vi "I am alive.vi"(8 "error in (no error)":errorcluster, 11 "Guardian in":refnum<class "Guardian.lvclass">) -> (0 "error out":errorcluster, 3 "Guardian out":refnum<class "Guardian.lvclass">)   [LabVIEW 2026, in "TALOS.lvlib" / "Guardian.lvlib" / "Guardian.lvclass"]
doc: "This VI updates the Guardian Health SV, indicating the Guardian is working properly to the other Guardians."
uses:
  Guardian.lvclass
  C:/LabVIEW Code/TALOS/builds/Actor Framework PPL/Actor Framework.lvlibp/1abvi3w/vi.lib/ActorFramework/Actor/Actor.lvclass
  C:/LabVIEW Code/TALOS/talos/Ancestor/Ancestor/Ancestor.lvclass
  Guardian.lvclass/Guardian.ctl
  Ancestor/Ancestor/Ancestor.lvclass/Ancestor.ctl
  Guardian Messages/Message to Other Guardian Msg/Message to Other Guardian Msg.lvclass/Message to Other Guardian Msg.ctl
  Guardian Messages/TCP-SV Message Interpreter Msg/TCP-SV Message Interpreter Msg.lvclass/TCP-SV Message Interpreter Msg.ctl
  Guardian Messages/Message to Other Guardian Msg/Send Message to Other Guardian.vi
  Ancestor/Ancestor/Read ID.vi
  Support VIs/Search Array of Strings.vi
  Guardian Messages/TCP-SV Message Interpreter Msg/Send TCP-SV Message Interpreter.vi
  Support VIs/Substitute Error.vi
  Support VIs/Generate Error.vi
  FGV/Error Memory/Get Error Description.vi
  Support VIs/Get PC name.vi
  Support VIs/Get Class Name.vi
  <vilib>/Utility/error.llb/Clear Errors.vi
  FGV/Error Memory/Error Memory Core.vi
  <vilib>/AdvancedString/Delimited String to 1D String Array.vi
  <vilib>/AdvancedString/Delimited String to 1D String Array (string).vi
  Support VIs/Circus Root Path.vi
  FGV/Error Memory/Error Crt Lvl checker.vi
  FGV/Error Memory/Error Memory Core.vi/40c8088d-b597-4017-91af-faa98e00292e.vi
  FGV/Error Memory/Error Memory Core.vi/d4a3ab98-063c-4e44-b43d-fbdcfe6c2be2.vi
  Support VIs/Global Constants.vi
  Support VIs/Circus Critical PCs List.vi
  builds/Actor Framework PPL/Actor Framework.lvlibp/1abvi3w/vi.lib/ActorFramework/Actor/Read Self Enqueuer.vi
  builds/Actor Framework PPL/Actor Framework.lvlibp/1abvi3w/vi.lib/ActorFramework/Message Enqueuer/Enqueue.vi
  Support VIs/Global Memory.vi
  <vilib>/Utility/LVClass/Get LV Class Name.vi
  Support VIs/Is in Packed Library.vi
  Support VIs/TALOS Root path.vi
  Support VIs/Read CSV worksheet.vi
  <vilib>/Utility/error.llb/General Error Handler.vi
  Support VIs/Error Log.vi
  Guardian Messages/Message to Other Guardian Msg/Message to Other Guardian Msg.lvclass
  Guardian Messages/TCP-SV Message Interpreter Msg/TCP-SV Message Interpreter Msg.lvclass
  Ancestor/Ancestor/Ancestor.lvclass
  <vilib>/Comparison/Equal/Equal Functor/Equal Functor.lvclass
  Classes/Guardian List/Guardian List.lvclass
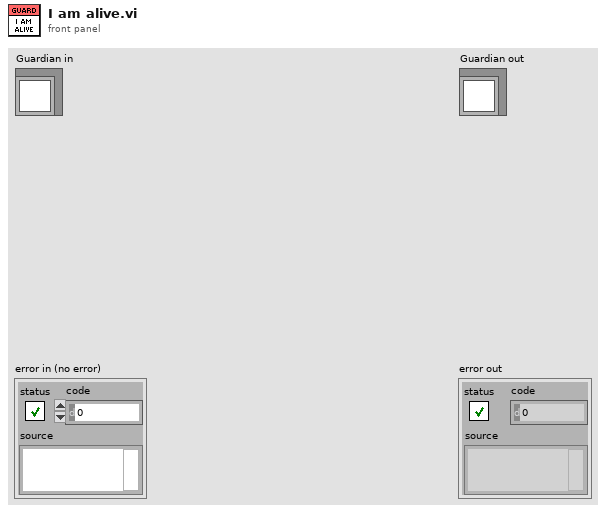
[diagram p1: front panel]
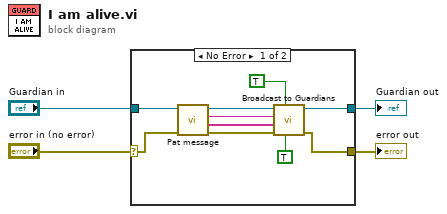
[diagram p0: block diagram]
diagram:
  n1 = case shown="No Error" "error in (no error)" {
    selector: "error in (no error)" -> [w13 w16]
    tunnel: [w8 w16] -> w3
    tunnel: [w9 w15] -> w1
    tunnel: "Guardian in" -> [w14 w15]
    frame No Error {
      n2 = call "Pat message.vi"("error in (no error)"=w13, "Guardian in"=w14) -> ("error out"=w11:errorcluster, "Data"=w10:string[], "Message name"=w6:string, "Guardian out"=w12:refnum<class "Guardian.lvclass">)  [unwired: 6 in]
      n3 = call "Broadcast to Guardians.vi"("Only active ones?"=TRUE, "Local also?"=TRUE, "error in (no error)"=w11, "Data"=w10, "Message"=w6, "Guardian in"=w12) -> ("error out"=w8:errorcluster, "Guardian out"=w9:refnum<class "Guardian.lvclass">)  [unwired: 4 in]
    }
    frame Error {
    }
  }
  "error out" <- w3
  "Guardian out" <- w1
